vi "GetDoubleTaskVariable.vi"(8 "error in":errorcluster, 9 "varNumber":i32, 10 "taskId":i32(ring) items=["TLibrary", "T01", "T02", "T03", "T04", "T05", "T06", "T07", "T08", "T09", "T10", "T11", "T12", "T13", "T14", "T15", "T16", "T17", "T18", "T19", "T20", "T21", "T22", "T23", "T24", "T25", "T26", "T27", "T28", "T29", "T30", "T31"], 11 "controller in":refnum<k24>) -> (0 "error out":errorcluster, 2 "double variable out":dbl, 3 "controller out":refnum<k24>)   [LabVIEW 2010]
uses:
  c:/aerotech/controller/dev/A3200/pc/labview/2010/bin/Aerotech.A3200.dll
  bin/Aerotech.A3200.dll
  c:/aerotech/controller/dev/A3200/pc/labview/2010/bin/Aerotech.A3200.LabVIEW.dll
  bin/Aerotech.A3200.LabVIEW.dll
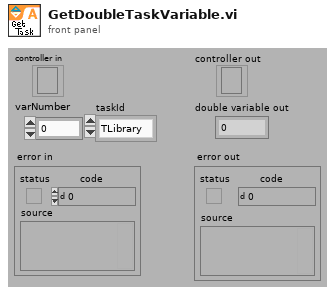
[diagram p1: front panel]
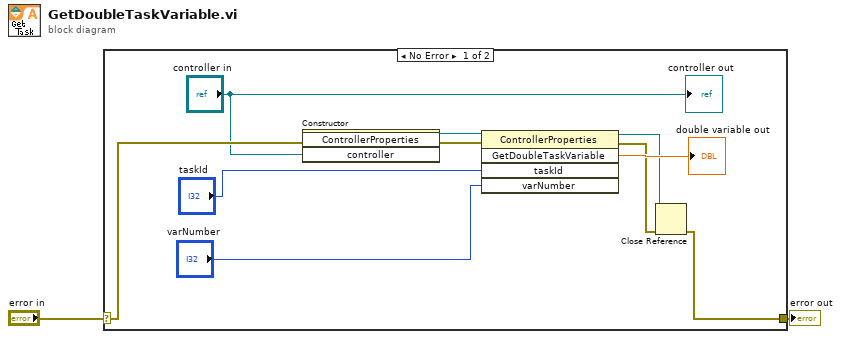
[diagram p0: block diagram]
diagram:
  n1 = case shown="No Error" "error in" {
    selector: "error in" -> [w12 w13]
    tunnel: [w3 w13] -> w1
    frame No Error {
      n2 = constructor class="ControllerProperties"(error in=w12, "controller"="controller in") -> (reference out=w11:refnum<k24>, error out=w10:errorcluster)  [unwired: 2 in, 2 out]
      n3 = invoke class="ControllerProperties" method="GetDoubleTaskVariable"(reference=w11, error in=w10, "taskId"="taskId", "varNumber"="varNumber") -> (reference out=w4:refnum<k24>, error out=w5:errorcluster, "GetDoubleTaskVariable"=→"double variable out":dbl)  [unwired: 1 in, 2 out]
      n4 = Close Reference(reference=w4, error in (no error)=w5) -> (error out=w3:errorcluster)
      "controller out" <- "controller in"
    }
    frame Error {
    }
  }
  "error out" <- w1
